vi "Get Sensor File Path.vi"(8 "error in (no error)":errorcluster, 10 "Test Channel Map":variant, 11 "Sensor Parameter in":refnum<class "Sensor Parameter.lvclass">) -> (0 "error out":errorcluster, 2 "Sensor File Path":path, 3 "Sensor Parameter out":refnum<class "Sensor Parameter.lvclass">)   [LabVIEW 2013, in "Parameter.lvlib" / "Sensor Parameter.lvclass"]
uses:
  Sensor Parameter.lvclass
  Abstract Sensor Parameter/Abstract Sensor Parameter.lvclass/Abstract Sensor Parameter.ctl
  Abstract Sensor Parameter/Data Accessors/Get Node Name.vi
  Abstract Sensor Parameter/Data Accessors/Get Channel Name.vi
  <vilib>/xml/Load XML File.vi
  <vilib>/xml/Close Reference(Node).vi
  <vilib>/xml/NI_XML.lvlib
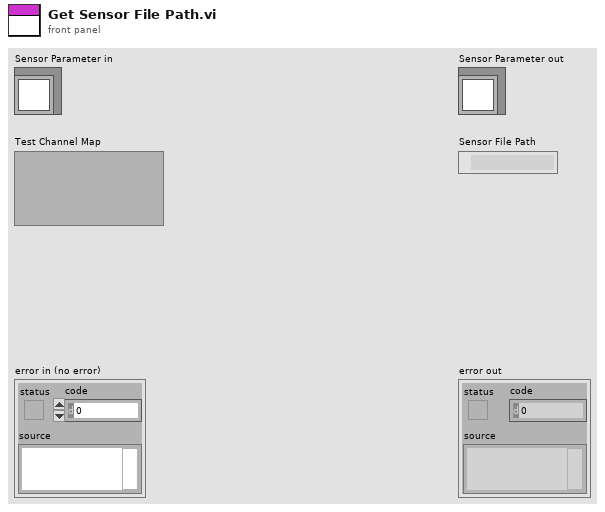
[diagram p1: front panel]
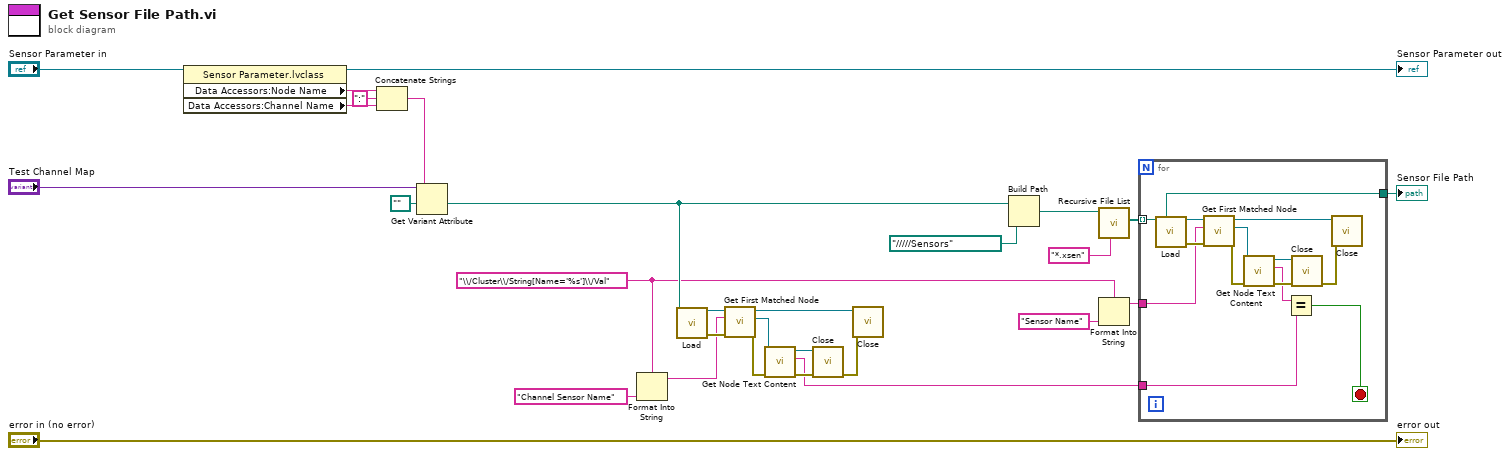
[diagram p0: block diagram]
diagram:
  w5 = "\\/Cluster\\/String[Name='%s']\\/Val" ("XPath expression")
  n1 = property class="Sensor Parameter.lvclass"(reference="Sensor Parameter in") -> (reference out=→"Sensor Parameter out":refnum<class "Sensor Parameter.lvclass">, "Data Accessors:Node Name"=w26:string, "Data Accessors:Channel Name"=w25:string)  [unwired: 1 in, 1 out]
  n2 = Concatenate Strings(w26, ":" ("string"), w25) -> (w22:string)
  n3 = Get Variant Attribute(Variant="Test Channel Map", name=w22, default value (empty Variant)=path "") -> (value=w10:path)  [unwired: 1 in, 3 out]
  n4 = Format Into String(format string=w5, "Channel Sensor Name" ("input 1")) -> (resulting string=w11:string)  [unwired: 2 in, 1 out]
  n5 = call-poly <vilib>:"Load.vi"("path to XML document"=w10) -> ("DOM document out"=w17:refnum<k20>, "error out"=w13:errorcluster)  [unwired: 12 in, 1 out]
  n6 = call <vilib>:"Get First Matched Node.vi"("error in (no error)"=w13, "XPath expression"=w11, "node in"=w17) -> ("error out"=w19:errorcluster, "node result"=w20:refnum<k20>, "node out"=w15:refnum<k20>)  [unwired: 6 in]
  n7 = call <vilib>:"Get Node Text Content.vi"("error in (no error)"=w19, "node in"=w20) -> ("error out"=w16:errorcluster, "node text"=w2:string, "node out"=w18:refnum<k20>)  [unwired: 7 in]
  n8 = call-poly <vilib>:"Close.vi"("error in (no error)"=w16, "node"=w18) -> ("error out"=w14:errorcluster)  [unwired: 7 in]
  n9 = call-poly <vilib>:"Close.vi"("error in (no error)"=w14, "node"=w15) -> ()  [unwired: 7 in, 1 out]
  n10 = Build Path(base path=w10, name or relative path=path "../../../../../Sensors") -> (appended path=w8:path)
  n11 = call <vilib>:"Recursive File List.vi"("pattern"="*.xsen", "Folder Path"=w8) -> ("All Files in Dir"=w6:path[])  [unwired: 5 in, 4 out]
  n12 = Format Into String(format string=w5, "Sensor Name" ("input 1")) -> (resulting string=w3:string)  [unwired: 2 in, 1 out]
  n13 = for {
    tunnel: w6 -> [w30] mode=indexing
    tunnel: w3 -> [w34]
    tunnel: w2 -> [w32]
    tunnel: [w30] -> w1
    stop <- w31 stop-if-true
    n14 = call-poly <vilib>:"Load.vi"("path to XML document"=w30) -> ("DOM document out"=w39:refnum<k20>, "error out"=w35:errorcluster)  [unwired: 12 in, 1 out]
    n15 = call <vilib>:"Get First Matched Node.vi"("error in (no error)"=w35, "XPath expression"=w34, "node in"=w39) -> ("error out"=w41:errorcluster, "node result"=w42:refnum<k20>, "node out"=w37:refnum<k20>)  [unwired: 6 in]
    n16 = call <vilib>:"Get Node Text Content.vi"("error in (no error)"=w41, "node in"=w42) -> ("error out"=w38:errorcluster, "node text"=w33:string, "node out"=w40:refnum<k20>)  [unwired: 7 in]
    n17 = Equal?(x=w33, y=w32) -> (x = y?=w31:bool)
    n18 = call-poly <vilib>:"Close.vi"("error in (no error)"=w38, "node"=w40) -> ("error out"=w36:errorcluster)  [unwired: 7 in]
    n19 = call-poly <vilib>:"Close.vi"("error in (no error)"=w36, "node"=w37) -> ()  [unwired: 7 in, 1 out]
  }
  "Sensor File Path" <- w1
  "error out" <- "error in (no error)"
